vi "Close.vi"(8 "Error In":errorcluster, 11 "IScope in":refnum<class "IRead Waveform.lvclass">) -> (0 "Error Out":errorcluster, 3 "IScope out":refnum<class "IRead Waveform.lvclass">)   [LabVIEW 2023, in "HAL Interfaces.lvlib" / "IRead Waveform.lvclass"]
uses:
  IRead Waveform.lvclass
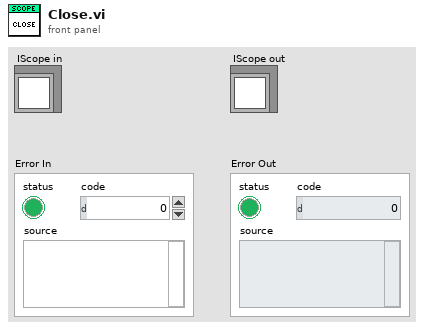
[diagram p1: front panel]
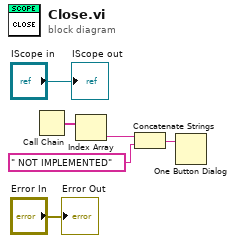
[diagram p0: block diagram]
diagram:
  n1 = Call Chain() -> (call chain=w4:string[])
  n2 = Index Array(array=w4) -> (element=w2:string)  [unwired: 1 in]
  n3 = Concatenate Strings(w2, " NOT IMPLEMENTED" ("string")) -> (w3:string)
  n4 = One Button Dialog(message=w3) -> ()  [unwired: 1 in, 1 out]
  "Error Out" <- "Error In"
  "IScope out" <- "IScope in"
